vi "CTD_to_Data.vi"(1 "CommonTargetData":T2) -> (0 "Data":T1)   [LabVIEW 2011]
uses:
  CommonTargetData.ctl
  TargetData.ctl
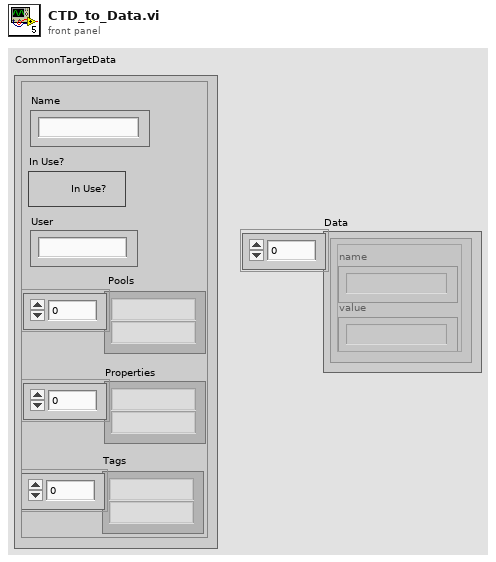
[diagram p1: front panel]
types:
  T1 = typedef "TargetData.ctl" = cluster{"name":string, "value":string}[]
  T2 = typedef "CommonTargetData.ctl" = cluster{"Name":string, "In Use?":bool, "User":string, " Pools":string[], "Tags":string[], "Properties":string[]}
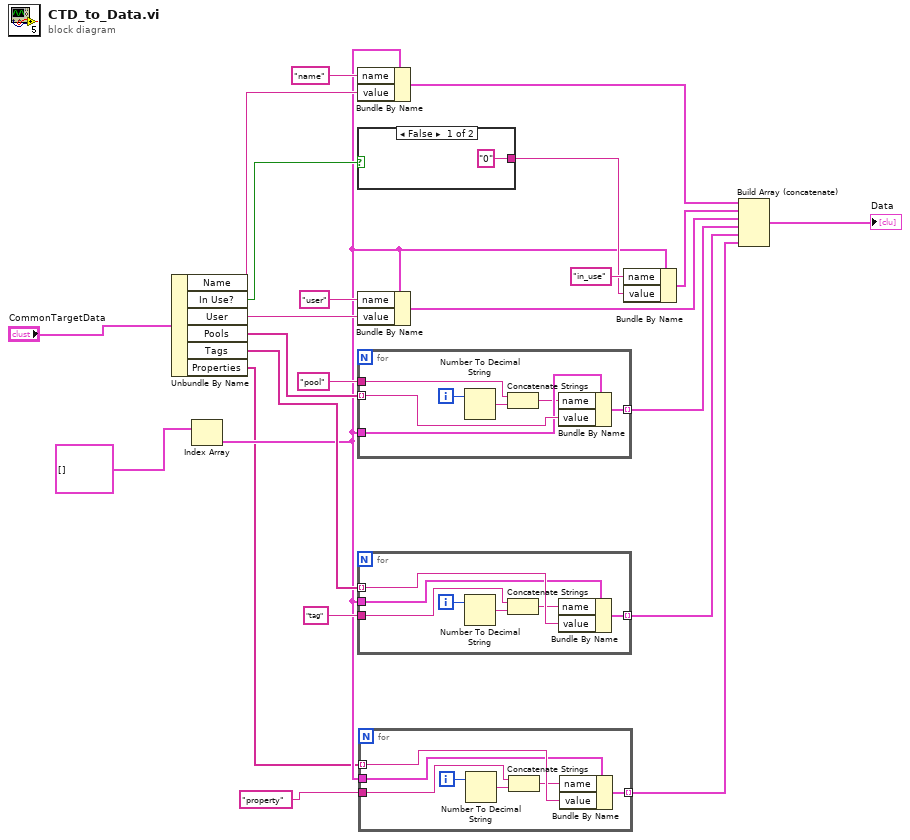
[diagram p0: block diagram]
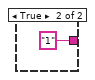
[diagram p2: hidden frame]
diagram:
  n1 = Unbundle By Name("CommonTargetData") -> ("Name"=w15:string, "In Use?"=w14:bool, "User"=w13:string, "Pools"=w11:string[], "Tags"=w8:string[], "Properties"=w3:string[])
  n2 = Index Array(array=T1 [] ("Data")) -> (element=w4:cluster{"name":string, "value":string})  [unwired: 1 in]
  n3 = Bundle By Name(cluster=w4, "name"="name", "value"=w15) -> (w23:cluster{"name":string, "value":string})
  n4 = case shown="False" w14 {
    tunnel: ["0" ("value") "1" ("value")] -> w17
    frame False {
    }
    frame True {
    }
  }
  n5 = Bundle By Name(cluster=w4, "name"="user", "value"=w13) -> (w18:cluster{"name":string, "value":string})
  n6 = for {
    tunnel: "pool" ("name") -> [w30]
    tunnel: w11 -> [w32] mode=indexing
    tunnel: w4 -> [w31]
    tunnel: [w26] -> w10 mode=indexing
    i -> [w29]
    n7 = Number To Decimal String(number=w29) -> (decimal integer string=w28:string)  [unwired: 1 in]
    n8 = Concatenate Strings(w30, w28) -> (w27:string)
    n9 = Bundle By Name(cluster=w31, "name"=w27, "value"=w32) -> (w26:cluster{"name":string, "value":string})
  }
  n10 = for {
    tunnel: "tag" ("name") -> [w37]
    tunnel: w8 -> [w39] mode=indexing
    tunnel: w4 -> [w38]
    tunnel: [w33] -> w7 mode=indexing
    i -> [w36]
    n11 = Number To Decimal String(number=w36) -> (decimal integer string=w35:string)  [unwired: 1 in]
    n12 = Concatenate Strings(w37, w35) -> (w34:string)
    n13 = Bundle By Name(cluster=w38, "name"=w34, "value"=w39) -> (w33:cluster{"name":string, "value":string})
  }
  n14 = for {
    tunnel: "property" ("name") -> [w44]
    tunnel: w3 -> [w46] mode=indexing
    tunnel: w4 -> [w45]
    tunnel: [w40] -> w5 mode=indexing
    i -> [w43]
    n15 = Number To Decimal String(number=w43) -> (decimal integer string=w42:string)  [unwired: 1 in]
    n16 = Concatenate Strings(w44, w42) -> (w41:string)
    n17 = Bundle By Name(cluster=w45, "name"=w41, "value"=w46) -> (w40:cluster{"name":string, "value":string})
  }
  n18 = Bundle By Name(cluster=w4, "name"="in_use", "value"=w17) -> (w19:cluster{"name":string, "value":string})
  n19 = Build Array (concatenate)(w23, w19, w18, w10, w7, w5) -> (→"Data":cluster{"name":string, "value":string}[])
